vi "Replace File Name.vi"(8 "error in (no error)":errorcluster, 10 "Actigraph ID":i32, 11 "Binary Data":u8[](array[numeric])) -> (0 "error out":errorcluster, 3 "File Name":string)   [LabVIEW 2019]
uses:
  Controls/gyro_control_time_informations.ctl
  Controls/gyro_control_memory_structure.ctl
  Controls/gyro_control_measurement_settings.ctl
  Controls/gyro_control_measurement_data.ctl
  Controls/gyro_control_all_in_one_package.ctl
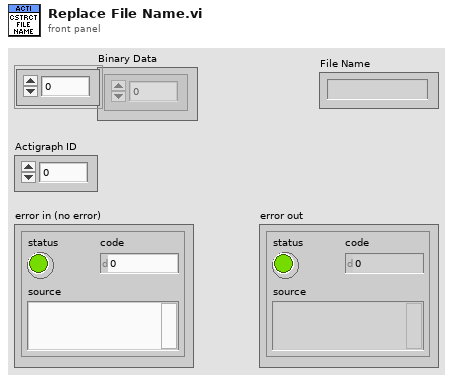
[diagram p1: front panel]
types:
  T1 = typedef "gyro_control_all_in_one_package.ctl" = cluster{"measurement data":T2, "actigraph settings":T3, "memory structure":T4, "time informations":T5}
  T2 = typedef "gyro_control_measurement_data.ctl" = cluster{"number of samples per axis":i32, "timestamp array":dbl[], "offset array":dbl[], "x, y, z axis data":waveform(dbl)[], "magnitude of acceleartion vectors":waveform(dbl), "statistics":cluster{"mean of x axis acceleration":dbl, "standard devation \nof x axis acceleration":dbl, "mean of y axis acceleration":dbl, "standard devation \nof y axis acceleration":dbl, "mean of z axis acceleration":dbl, "standard devation \nof z axis acceleration":dbl, "mean of magnitude\n of acceleration":dbl, "standard devation \nof magnitude of acceleration":dbl}, "voltage":waveform(dbl)}
  T3 = typedef "gyro_control_measurement_settings.ctl" = cluster{"# Pages":i32, "ODR":u8, "xlRange":u8, "gyroRange":u8, "id":u8, "Samplig Freq [Hz]":dbl, "xlRange in g":dbl, "gyroRange in dps":dbl}
  T4 = typedef "gyro_control_memory_structure.ctl" = cluster{"length of metadata [byte]":i32, "length of page [byte]":i32, "length of measurement \ndata on page [byte]":i32, "length of dataset [byte]":i32}
  T5 = typedef "gyro_control_time_informations.ctl" = cluster{"starting time":timestamp, "ending time":timestamp, "dt[s]":dbl, "sampling rate [Hz]":dbl, "length":dbl}
  T6 = typedef "control_all_in_one_package.ctl" = cluster{"memory structure":T7, "actigraph settings":T8, "time informations":T9, "measurement data":T10}
  T7 = typedef "control_memory_structure.ctl" = cluster{"length of metadata [byte]":i32, "length of page [byte]":i32, "length of measurement data on page [byte]":i32, "length of dataset [byte]":i32}
  T8 = typedef "control_measurement_settings.ctl" = cluster{"sampling frequency [Hz]":dbl, "measurement interval [± g]":i32, "high precision?":bool, "number of pages":i32, "rate code":i32, "range code":i32, "id":i32}
  T9 = typedef "control_time_informations.ctl" = cluster{"starting time":timestamp, "ending time":timestamp, "dt[s]":dbl, "sampling rate [Hz]":dbl, "length":dbl}
  T10 = typedef "control_measurement_data.ctl" = cluster{"number of samples per axis":i32, "timestamp array":dbl[], "offset array":dbl[], "x, y, z axis data":waveform(dbl)[], "normalised magnitude of acceleartion vectors":waveform(dbl), "calibration coefficients":T11, "statistics":T12, "battery voltage":waveform(dbl), "magnitude of acceleartion vectors":waveform(dbl)}
  T11 = typedef "control_calibration_coefficients.ctl" = cluster{"Sx":dbl, "Ox":dbl, "Sy":dbl, "Oy":dbl, "Sz":dbl, "Oz":dbl}
  T12 = typedef "control_statistics.ctl" = cluster{"mean of x axis acceleration":dbl, "standard devation of x axis acceleration":dbl, "mean of y axis acceleration":dbl, "standard devation of y axis acceleration":dbl, "mean of z axis acceleration":dbl, "standard devation of z axis acceleration":dbl, "mean of normalised magnitude of acceleration":dbl, "standard devation of normalised magnitude of acceleration":dbl}
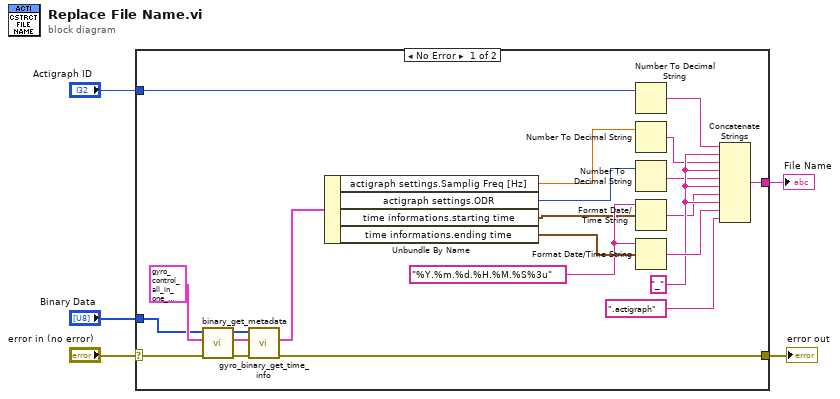
[diagram p0: block diagram]
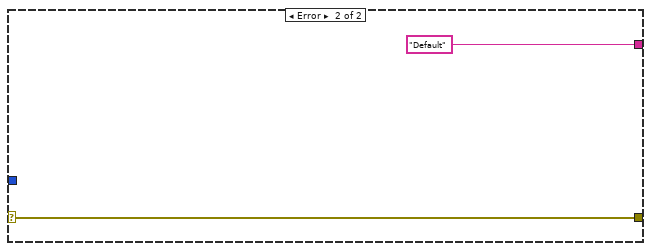
[diagram p2: hidden frame]
diagram:
  n1 = case shown="No Error" "error in (no error)" {
    selector: "error in (no error)" -> [w8 w29]
    tunnel: "Actigraph ID" -> [w27 _]
    tunnel: [w7 w29] -> w4
    tunnel: "Binary Data" -> [w9 _]
    tunnel: [w6 "Default"] -> w1
    frame No Error {
      w24 = "_"
      w16 = "%Y.%m.%d.%H.%M.%S%3u" ("time format string (%c)")
      n2 = call "binary_get_metadata.vi"("error in"=w8, "all in one package in"=T1 {"measurement data"={"number of samples per axis"=0, "timestamp array"=[], "offset array"=[], "x, y, z axis data"=[], "magnitude of acceleartion vectors"={"t0"=timestamp(0 s since 1904-01-01), "dt"=1.0, "Y"=[]}, "statistics"={"mean of x axis acceleration"=0.0, "standard devation \nof x axis acceleration"=0.0, "mean of y axis acceleration"=0.0, "standard devation \nof y axis acceleration"=0.0, "mean of z axis acceleration"=0.0, "standard devation \nof z axis acceleration"=0.0, "mean of magnitude\n of acceleration"=0.0, "standard devation \nof magnitude of acceleration"=0.0}, "voltage"={"t0"=timestamp(0 s since 1904-01-01), "dt"=1.0, "Y"=[]}}, "actigraph settings"={"# Pages"=0, "ODR"=0, "xlRange"=0, "gyroRange"=0, "id"=0, "Samplig Freq [Hz]"=0.0, "xlRange in g"=0.0, "gyroRange in dps"=0.0}, "memory structure"={"length of metadata [byte]"=5, "length of page [byte]"=2048, "length of measurement \ndata on page [byte]"=2028, "length of dataset [byte]"=6}, "time informations"={"starting time"=timestamp(0 s since 1904-01-01), "ending time"=timestamp(0 s since 1904-01-01), "dt[s]"=0.0, "sampling rate [Hz]"=0.0, "length"=0.0}}, "binary data w/ calibration coefficients"=w9) -> ("error out"=w11:errorcluster, "all in one package out"=w13:T6, "pages"=w12:u8[])  [unwired: 6 in]
      n3 = call "gyro_binary_get_time_info.vi"("error in"=w11, "all in one package in"=w13, "pages"=w12) -> ("error out"=w7:errorcluster, "all in one package out"=w14:T1)  [unwired: 6 in, 1 out]
      n4 = Unbundle By Name(w14) -> ("actigraph settings.Samplig Freq [Hz]"=w18:dbl, "actigraph settings.ODR"=w19:u8, "time informations.starting time"=w15:timestamp, "time informations.ending time"=w17:timestamp)
      n5 = Number To Decimal String(number=w27) -> (decimal integer string=w20:string)  [unwired: 1 in]
      n6 = Number To Decimal String(number=w18) -> (decimal integer string=w21:string)  [unwired: 1 in]
      n7 = Number To Decimal String(number=w19) -> (decimal integer string=w22:string)  [unwired: 1 in]
      n8 = Format Date/Time String(time format string (%c)=w16, seconds (now)=w15) -> (date/time string=w23:string)  [unwired: 1 in]
      n9 = Format Date/Time String(time format string (%c)=w16, seconds (now)=w17) -> (date/time string=w25:string)  [unwired: 1 in]
      n10 = Concatenate Strings(w20, w24, w21, w24, w22, w24, w23, w24, w25, ".actigraph") -> (w6:string)
    }
    frame Error {
    }
  }
  "error out" <- w4
  "File Name" <- w1
